vi "Functional Global - Individual Trial Parameters.vi"(7 "Method":T1, 8 "error in (no error)":errorcluster, 10 "Variable Name":string, 11 "connection ID":refnum<k5>) -> (0 "error out":errorcluster, 2 "Variable Value":string, 3 "connection ID (duplicate)":refnum<k5>)   [LabVIEW 2010, in "Core SubVIs.lvlib"]
uses:
  Core SubVIs.lvlib
  Controls/TYPE - Individual Trial Parameters Method.ctl
  Controls/TYPE - Configure Test Method.ctl
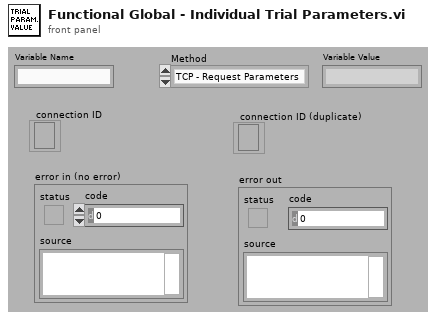
[diagram p1: front panel]
types:
  T1 = typedef "Core SubVIs.lvlib/TYPE - Individual Trial Parameters Method.ctl" = enum16{"TCP - Request Parameters", "Read Variable by Name"}
  T2 = enum16{"Standard", "Buffered", "CRLF", "Immediate"}
  T3 = typedef "Core SubVIs.lvlib/TYPE - Configure Test Method.ctl" = enum16{"Read Configuration", "Load Configuration from File", "Load from default file", "Configuration Dialog"}
  T4 = cluster{"Name":string, "Type":string, "value":string}[]
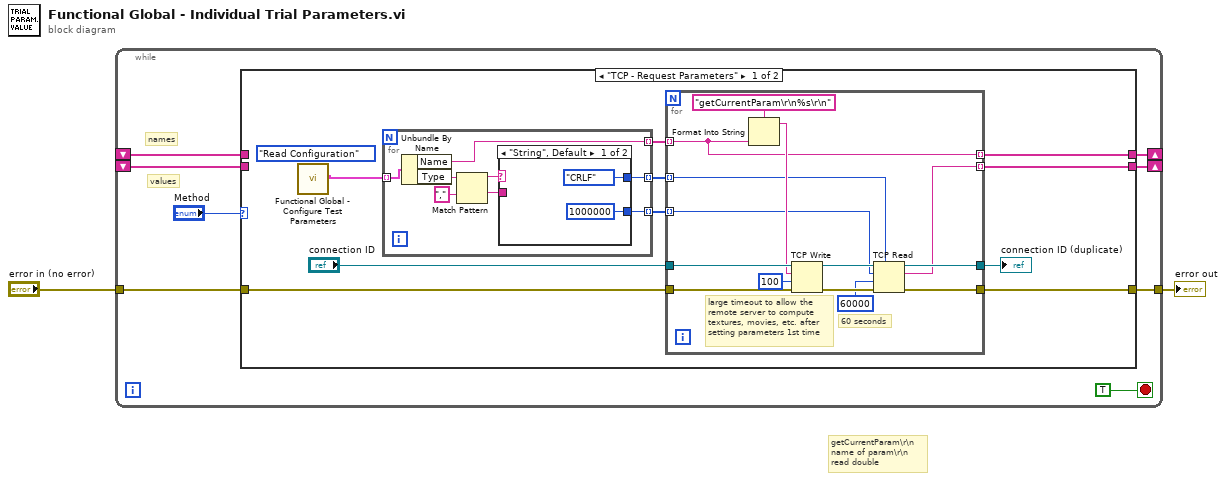
[diagram p0: block diagram]
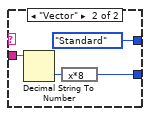
[diagram p2: hidden frame]
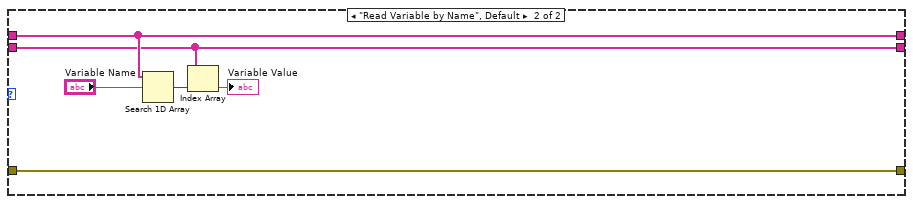
[diagram p3: hidden frame]
diagram:
  # "getCurrentParam\\r\\n\nname of param\\r\\n\nread double"
  n1 = while {
    tunnel: [w10] -> w2
    tunnel: "error in (no error)" -> [w9]
    shift-right: [w7] -> _
    shift-left: _ -> [w4]
    shift-right: [w6] -> _
    shift-left: _ -> [w5]
    stop <- TRUE stop-if-true
    # "values"
    # "names"
    n2 = case shown="\"TCP - Request Parameters\"" "Method" {
      tunnel: [w20 w49] -> w10
      tunnel: w9 -> [w19 w49]
      tunnel: [w14 w51] -> w7
      tunnel: [w13 w54] -> w6
      tunnel: w5 -> [_ w54]
      tunnel: w4 -> [_ w51]
      frame "TCP - Request Parameters" {
        (unwired) TYPE_-_Configure_Test_Method."Read Configuration" ("Configure Test Method")
        n3 = call "Functional Global - Configure Test Parameters.vi"() -> ("Experiment Parameter Values"=w11:T4)  [unwired: 10 in, 1 out]
        n4 = for {
          tunnel: w11 -> [w26] mode=indexing
          tunnel: [w23] -> w15 mode=indexing
          tunnel: [w22] -> w16 mode=indexing
          tunnel: [w21] -> w12 mode=indexing
          n5 = Unbundle By Name(w26) -> ("Name"=w22:string, "Type"=w28:string)
          n6 = Match Pattern(string=w28, regular expression=",") -> (before substring=w25:string, after substring=w24:string)  [unwired: 1 in, 2 out]
          n7 = case shown="\"String\", Default" w25 {
            tunnel: w24 -> [_ w34]
            tunnel: [1000000 w32] -> w23
            tunnel: [T2."CRLF" ("mode (standard)") T2."Standard" ("mode (standard)")] -> w21
            frame "String", Default {
            }
            frame "Vector" {
              n8 = Decimal String To Number(string=w34) -> (number=w33:i32)  [unwired: 2 in, 1 out]
              n9 = expression code="x*8"(w33) -> (w32:i32)
            }
          }
        }
        n10 = for {
          tunnel: "connection ID" -> [w48]
          tunnel: w19 -> [w47]
          tunnel: [w39] -> w18
          tunnel: [w38] -> w20
          tunnel: w16 -> [w36] mode=indexing
          tunnel: w15 -> [w40] mode=indexing
          tunnel: [w37] -> w14 mode=indexing
          tunnel: [w36] -> w13 mode=indexing
          tunnel: w12 -> [w35] mode=indexing
          # "60 seconds"
          # "large timeout to allow the remote server to compute textures, movies, etc. after setting parameters 1st time"
          n11 = Format Into String(format string="getCurrentParam\r\n%s\r\n", w36) -> (resulting string=w45:string)  [unwired: 2 in, 1 out]
          n12 = TCP Write(connection ID=w48, data in=w45, error in (no error)=w47, 9:100 ("timeout ms (25000)")) -> (connection ID out=w43:refnum<k5>, error out=w42:errorcluster)  [unwired: 1 out]
          n13 = TCP Read(connection ID=w43, bytes to read=w40, error in (no error)=w42, 7:w35, 9:60000 ("timeout ms (25000)")) -> (connection ID out=w39:refnum<k5>, data out=w37:string, error out=w38:errorcluster)
        }
        "connection ID (duplicate)" <- w18
      }
      frame "Read Variable by Name", Default {
        n14 = Search 1D Array(1D array=w54, element="Variable Name") -> (index of element=w52:i32)  [unwired: 1 in]
        n15 = Index Array(array=w51, index=w52) -> (element=→"Variable Value":string)
      }
    }
  }
  "error out" <- w2
